vi "AK8963-self-test.vi"(8 "error in (no error)":errorcluster, 10 "ASA":u8[](array[numeric]), 11 "I2C Ref In":T1={"myRIO Reference"={"myRIO Model"=enum."Unknown", "myRIO Hardware Reference"={"Generic FPGA Reference"=refnum, "Allow multiple opens"=FALSE}}, "I2C Channels Enum"=enum."Not Connected", "I2C Configuration"={"I2C Transfer Rate"=enum."Fast mode (400 kbps)"}}) -> (0 "error out":errorcluster, 1 "Self-test":dbl[](array[numeric]), 3 "I2C Ref Out":T1={"myRIO Reference"={"myRIO Model"=enum."Unknown", "myRIO Hardware Reference"={"Generic FPGA Reference"=refnum, "Allow multiple opens"=FALSE}}, "I2C Channels Enum"=enum."Not Connected", "I2C Configuration"={"I2C Transfer Rate"=enum."Fast mode (400 kbps)"}})   [LabVIEW 2019]
uses:
  <vilib>/myRIO/Instrument Drivers/Onboard IO/I2C/typedefs/I2C Reference.ctl
  <vilib>/myRIO/Common/Instrument Driver Framework/Utilities/typedefs/myRIO Generic Hardware Reference.ctl
  <vilib>/myRIO/Common/Instrument Driver Framework/Utilities/typedefs/Hardware Version Enum.ctl
  <vilib>/myRIO/Common/Instrument Driver Framework/Utilities/typedefs/myRIO v1.0 Reference.ctl
  <vilib>/myRIO/Common/Instrument Driver Framework/Utilities/typedefs/Generic FPGA Reference.ctl
  <vilib>/myRIO/Common/Instrument Driver Framework/myRIO v1.0/I2C/typedefs/I2C Channels Enum.ctl
  <vilib>/myRIO/Instrument Drivers/Onboard IO/I2C/typedefs/I2C Configuration.ctl
  <vilib>/myRIO/Instrument Drivers/Onboard IO/I2C/typedefs/I2C Transfer Rate.ctl
  <vilib>/Utility/error.llb/Error Cluster From Error Code.vi
  <vilib>/myRIO/Common/Instrument Driver Framework/myRIO v1.0/I2C/vis/myRIO v1.0 Write I2C.vi
  <vilib>/myRIO/Common/Instrument Driver Framework/myRIO v1.0/I2C/vis/myRIO v1.0 Read I2C.vi
  <vilib>/ErrorRing/Error Ring.xnode
  <vilib>/myRIO/Instrument Drivers/Onboard IO/I2C/I2C.lvlib
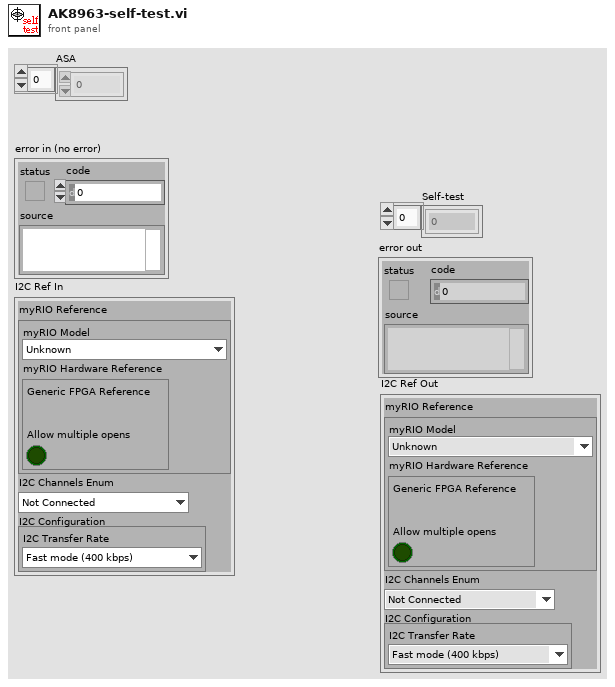
[diagram p1: front panel]
types:
  T1 = typedef "I2C.lvlib/I2C Reference.ctl" = cluster{"myRIO Reference":T2, "I2C Channels Enum":T6, "I2C Configuration":T7}
  T2 = typedef "myRIO Generic Hardware Reference.ctl" = cluster{"myRIO Model":T3, "myRIO Hardware Reference":T4}
  T3 = typedef "Hardware Version Enum.ctl" = enum16{"Unknown", "myRIO-1900", "myRIO-1950", "roboRIO", "NI ELVIS RIO CM", "ELVIS III"}
  T4 = typedef "myRIO v1.0 Reference.ctl" = cluster{"Generic FPGA Reference":T5, "Allow multiple opens":bool}
  T5 = typedef "Generic FPGA Reference.ctl" = refnum<k20>
  T6 = typedef "I2C Channels Enum.ctl" = enum16{"Not Connected", "A/I2C", "B/I2C", "I2C/I2C"}
  T7 = typedef "I2C.lvlib/I2C Configuration.ctl" = cluster{"I2C Transfer Rate":T8}
  T8 = typedef "I2C.lvlib/I2C Transfer Rate.ctl" = enum16{"Standard mode (100 kbps)", "Fast mode (400 kbps)"}
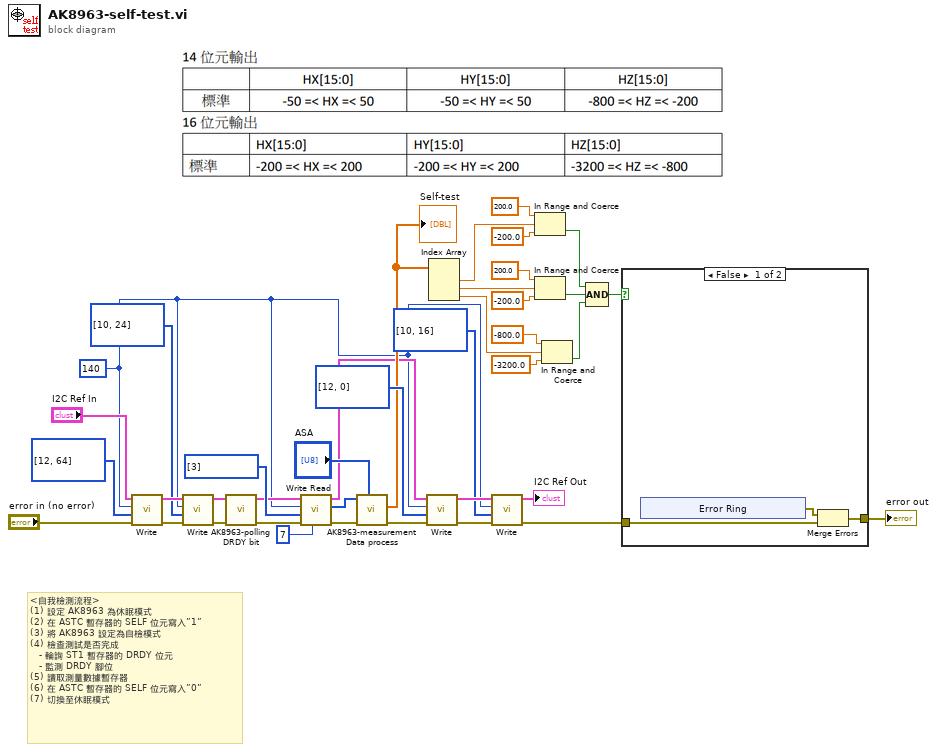
[diagram p0: block diagram]
diagram:
  w1 = u8 140 ("Slave Address (7-bit)")
  # "<自我檢測流程>\n(1) 設定 AK8963 為休眠模式\n(2) 在 ASTC 暫存器的 SELF 位元寫入”1”\n(3) 將 AK8963 設定為自檢模式\n(4) 檢查測試是否完成\n   - 輪詢 ST1 暫存器的 DRDY 位元\n   - 監測 DRDY 腳位\n(5) 讀取測量數據暫存器\n(6) 在 ASTC 暫存器的 SELF 位元寫入”0”\n(7) 切換至休眠模式"
  n1 = call <vilib>:"Write.vi"("error in (no error)"="error in (no error)", "Bytes to Write"=u8[] [12, 64], "Slave Address (7-bit)"=w1, "I2C Ref In"="I2C Ref In") -> ("error out"=w13:errorcluster, "I2C Ref Out"=w36:T1)  [unwired: 6 in]
  n2 = call <vilib>:"Write.vi"("error in (no error)"=w13, "Bytes to Write"=u8[] [10, 24], "Slave Address (7-bit)"=w1, "I2C Ref In"=w36) -> ("error out"=w11:errorcluster, "I2C Ref Out"=w12:T1)  [unwired: 6 in]
  n3 = call "AK8963-polling DRDY bit.vi"("error in"=w11, "I2C Ref in"=w12) -> ("error out 2"=w10:errorcluster, "I2C Ref Out 2"=w9:T1)  [unwired: 8 in]
  n4 = call <vilib>:"Write Read.vi"("Byte Count"=u32 7, "error in (no error)"=w10, "Bytes to Write"=u8[] [3], "Slave Address (7-bit)"=w1, "I2C Ref In"=w9) -> ("error out"=w8:errorcluster, "Bytes Read"=w7:u8[], "I2C Ref Out"=w3:T1)  [unwired: 3 in]
  n5 = call "AK8963-measurement Data process.vi"("ASA"="ASA", "error in"=w8, "Bytes Read"=w7) -> ("error OUT"=w5:errorcluster, "measure"=w4:dbl[])  [unwired: 7 in]
  "Self-test" <- w4
  n6 = call <vilib>:"Write.vi"("error in (no error)"=w5, "Bytes to Write"=u8[] [12, 0], "Slave Address (7-bit)"=w1, "I2C Ref In"=w3) -> ("error out"=w31:errorcluster, "I2C Ref Out"=w32:T1)  [unwired: 6 in]
  n7 = Index Array(array=w4) -> (element #1=w25:dbl, element #2=w22:dbl, element #3=w19:dbl)  [unwired: 3 in]
  n8 = call <vilib>:"Write.vi"("error in (no error)"=w31, "Bytes to Write"=u8[] [10, 16], "Slave Address (7-bit)"=w1, "I2C Ref In"=w32) -> ("error out"=w14:errorcluster, "I2C Ref Out"=→"I2C Ref Out":T1)  [unwired: 6 in]
  n9 = In Range and Coerce(upper limit=200.0, x=w25, lower limit=-200.0) -> (In Range?=w17:bool)  [unwired: 1 out]
  n10 = In Range and Coerce(upper limit=200.0, x=w22, lower limit=-200.0) -> (In Range?=w16:bool)  [unwired: 1 out]
  n11 = In Range and Coerce(upper limit=-800.0, x=w19, lower limit=-3200.0) -> (In Range?=w18:bool)  [unwired: 1 out]
  n12 = Compound Arithmetic op=AND(w17, w16, w18) -> (w15:bool)
  n13 = case shown="False" w15 {
    tunnel: [w42 w48] -> w2
    tunnel: w14 -> [w40 w48]
    frame False {
      n14 = xnode "Error Ring"() -> ("error out"=w41:errorcluster)
      n15 = Merge Errors(w41, w40) -> (w42:errorcluster)
    }
    frame True {
    }
  }
  "error out" <- w2
